vi "Read Thermistor 2.vi"() -> ()   [LabVIEW 2020, in "Acquisition.lvlib"]
uses:
  Acquisition.lvlib
  <vilib>/ULx/Create Channel.llb/ULx Create Channel (AI-Voltage-Basic).vi
  <vilib>/ULx/Timing.llb/ULx Timing (Sample Clock).vi
  <vilib>/ULx/Read.llb/ULx Read (Analog DBL 1Chan 1Samp).vi
panel:
  in  "Time Target (s)":dbl=5.0
  in  "rate":dbl=1000.0
  in  "samples per channel":i32=1000
  in  "sample mode":i32(ring) items=["FiniteSamples", "ContinuousSamples"]
  in  "minimum value":dbl=-5.0
  in  "maximum value":dbl=5.0
  in  "physical channels":refnum<k21>
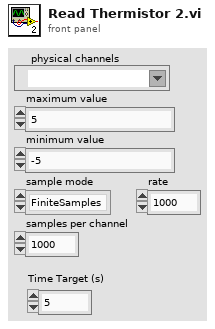
[diagram p1: front panel]
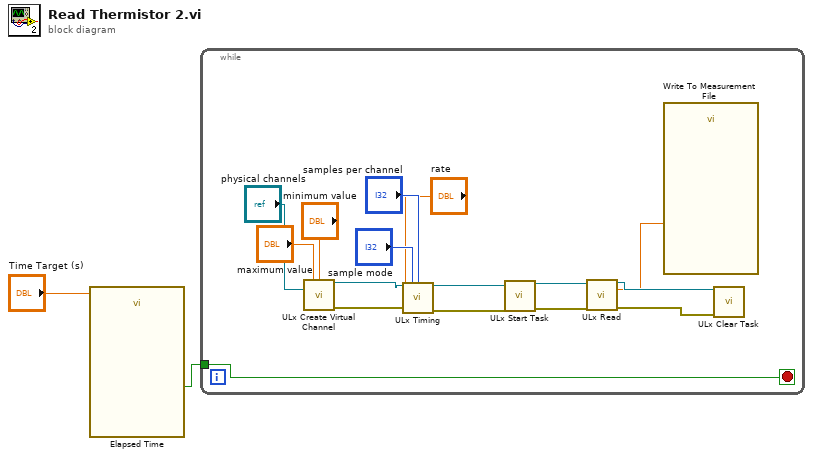
[diagram p0: block diagram]
diagram:
  n1 = call "Elapsed Time"("Time Target (s)"="Time Target (s)") -> ("Time has Elapsed"=w2:bool)  [unwired: 11 in, 7 out]
  n2 = while {
    tunnel: w2 -> [w3]
    stop <- w3 stop-if-true
    n3 = call-poly <vilib>:"ULx Create Virtual Channel.vi"("maximum value"="maximum value", "minimum value"="minimum value", "physical channels"="physical channels") -> ("task out"=w18:refnum<k24>, "error out"=w14:errorcluster)  [unwired: 11 in]
    n4 = call-poly <vilib>:"ULx Timing.vi"("task in"=w18, "sample mode"="sample mode", "samples per channel"="samples per channel", "rate"="rate", "error in"=w14) -> ("task out"=w17:refnum<k24>, "error out"=w13:errorcluster)  [unwired: 9 in]
    n5 = call <vilib>:"ULx Start Task.vi"("task in"=w17, "error in"=w13) -> ("task out"=w16:refnum<k24>, "error out"=w12:errorcluster)  [unwired: 12 in]
    n6 = call-poly <vilib>:"ULx Read.vi"("task in"=w16, "error in"=w12) -> ("task out"=w15:refnum<k24>, "data"=w4:dbl, "error out"=w11:errorcluster)  [unwired: 11 in]
    n7 = call "Write To Measurement File"("Signals"=w4) -> ()  [unwired: 16 in, 3 out]
    n8 = call <vilib>:"ULx Clear Task.vi"("task in"=w15, "error in"=w11) -> ()  [unwired: 13 in, 1 out]
  }
